vi "DrawMultiROI.vi"(8 "error in (no error)":errorcluster, 10 "ROIs":T2[](array[typedef]) {"Contours"."Type" items=["No Selection", "Point", "Line", "Rectangle", "Oval", "Polygon", "Freehand Region", "Annulus", "Unused2", "Unused3", "Broken Line", "Freehand Line", "Rotated Rectangle"]}, 11 "Image In":T1) -> (0 "error out":errorcluster, 3 "Image Out":T1)   [LabVIEW 2019]
uses:
  <vilib>/vision/Image Controls.llb/IMAQ Image.ctl
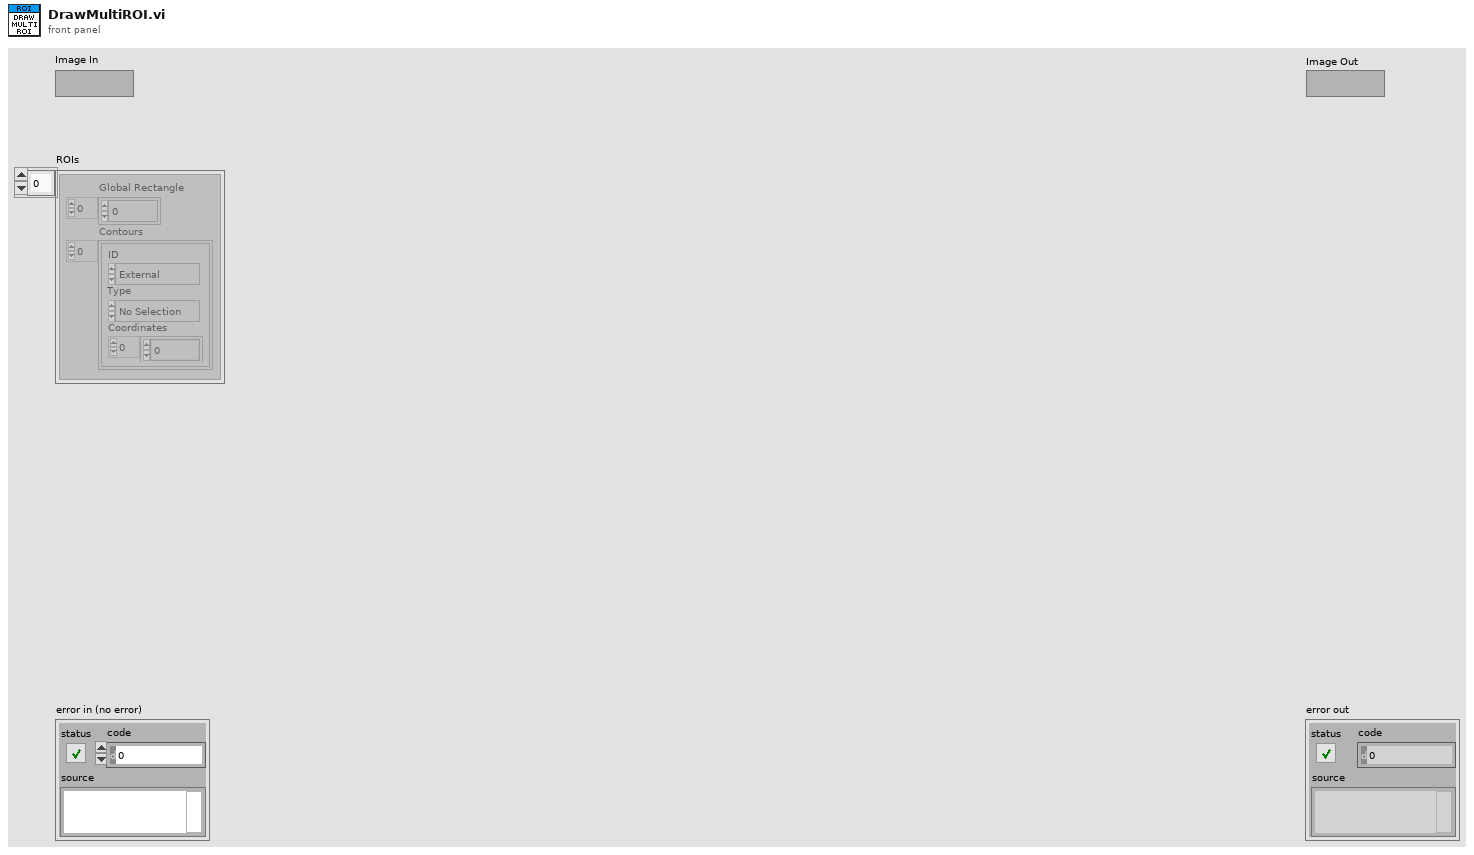
[diagram p1: front panel]
types:
  T1 = typedef "IMAQ Image.ctl" = refnum<image>
  T2 = typedef "ROI Descriptor" = cluster{"Global Rectangle":i32[], "Contours":cluster{"ID":enum32{"External", "Internal"}, "Type":u32, "Coordinates":i32[]}[]}
  T3 = cluster{"Desired Font (Application)":enum16{"User-specified Font", "Application Font", "System Font", "Dialog Font"}, "[User-specified Font]":cluster{"Font Name":string, "Size":i16, "Strikeout?":bool, "Italic?":bool, "Underline?":bool, "Outline?":bool, "Shadow?":bool, "Bold?":bool, "Rotation Angle":dbl}, "Horizontal Alignment":i16, "Vertical Alignment":i16}
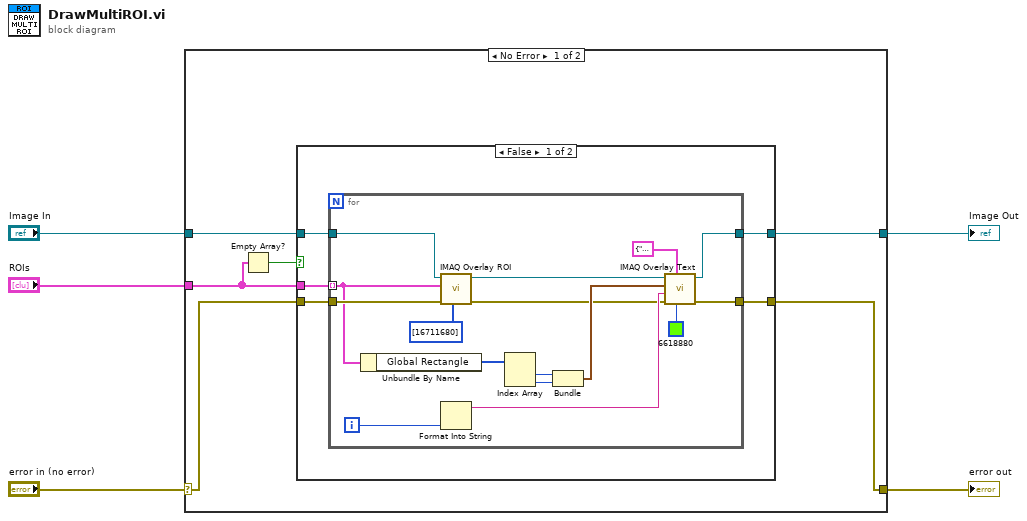
[diagram p0: block diagram]
diagram:
  n1 = case shown="No Error" "error in (no error)" {
    selector: "error in (no error)" -> [w11 w35]
    tunnel: "ROIs" -> [w6 _]
    tunnel: "Image In" -> [w10 w36]
    tunnel: [w9 w36] -> w2
    tunnel: [w8 w35] -> w1
    frame No Error {
      n2 = Empty Array?(array=w6) -> (empty?=w7:bool)
      n3 = case shown="False" w7 {
        tunnel: w6 -> [w16 _]
        tunnel: w11 -> [w15 w33]
        tunnel: w10 -> [w14 w34]
        tunnel: [w13 w34] -> w9
        tunnel: [w12 w33] -> w8
        frame False {
          n4 = for {
            tunnel: w15 -> [w31]
            tunnel: w16 -> [w30] mode=indexing
            tunnel: [w24] -> w13
            tunnel: w14 -> [w20]
            tunnel: [w19] -> w12
            i -> [w21]
            n5 = Unbundle By Name(w30) -> ("Global Rectangle"=w28:i32[])
            n6 = call "IMAQ Overlay ROI"("Colors (Green)"=u32[] [16711680], "error in (no error)"=w31, "ROI Descriptor"=w30, "Image"=w20) -> ("error out"=w17:errorcluster, "Image Out"=w29:T1)  [unwired: 6 in]
            n7 = Format Into String(w21) -> (resulting string=w22:string)  [unwired: 3 in, 1 out]
            n8 = Index Array(array=w28) -> (element #1=w27:i32, element #2=w26:i32)  [unwired: 2 in]
            n9 = Bundle(w27, w26) -> (w25:cluster{i32, i32})  [unwired: 1 in]
            n10 = call "IMAQ Overlay Text"("Text Color (black)"=u32 6618880, "Font, Size & Style"=T3 {"Desired Font (Application)"=enum."User-specified Font", "[User-specified Font]"={"Font Name"="", "Size"=18, "Strikeout?"=FALSE, "Italic?"=FALSE, "Underline?"=FALSE, "Outline?"=FALSE, "Shadow?"=FALSE, "Bold?"=FALSE, "Rotation Angle"=0.0}, "Horizontal Alignment"=0, "Vertical Alignment"=0}, "error in (no error)"=w17, "String"=w22, "Origin"=w25, "Image"=w29) -> ("error out"=w19:errorcluster, "Image Out"=w24:T1)  [unwired: 4 in]
          }
        }
        frame True {
        }
      }
    }
    frame Error {
    }
  }
  "error out" <- w1
  "Image Out" <- w2
